vi "Set Bucket Notification.vi"(8 "error in (no error)":errorcluster, 10 "Notification Configuration":T1, 11 "Bucket in":refnum<class "Bucket.lvclass">) -> (0 "error out":errorcluster, 2 "Test Message ID":string, 3 "Bucket out":refnum<class "Bucket.lvclass">)   [LabVIEW 2015, in "NI_AWS_S3.lvlib" / "Bucket.lvclass"]
uses:
  Bucket.lvclass
  Notification Configuration.ctl
  Topic Configuration.ctl
  Event.ctl
  Core/HTTP Request/Name Value Pair.ctl
  Cloud Function Configuration.ctl
  Queue Configuration.ctl
  Core/HTTP Request/Region handling.ctl
  Core/HTTP Request/Request Options.ctl
  Core/HTTP Request/URL formatting.ctl
  Bucket.lvclass/Bucket.ctl
  Read Name.vi
  <vilib>/regexp/Match Regular Expression.xnode
  Core/HTTP Request/HTTP Request.lvclass
  NI_AWS_S3.lvlib
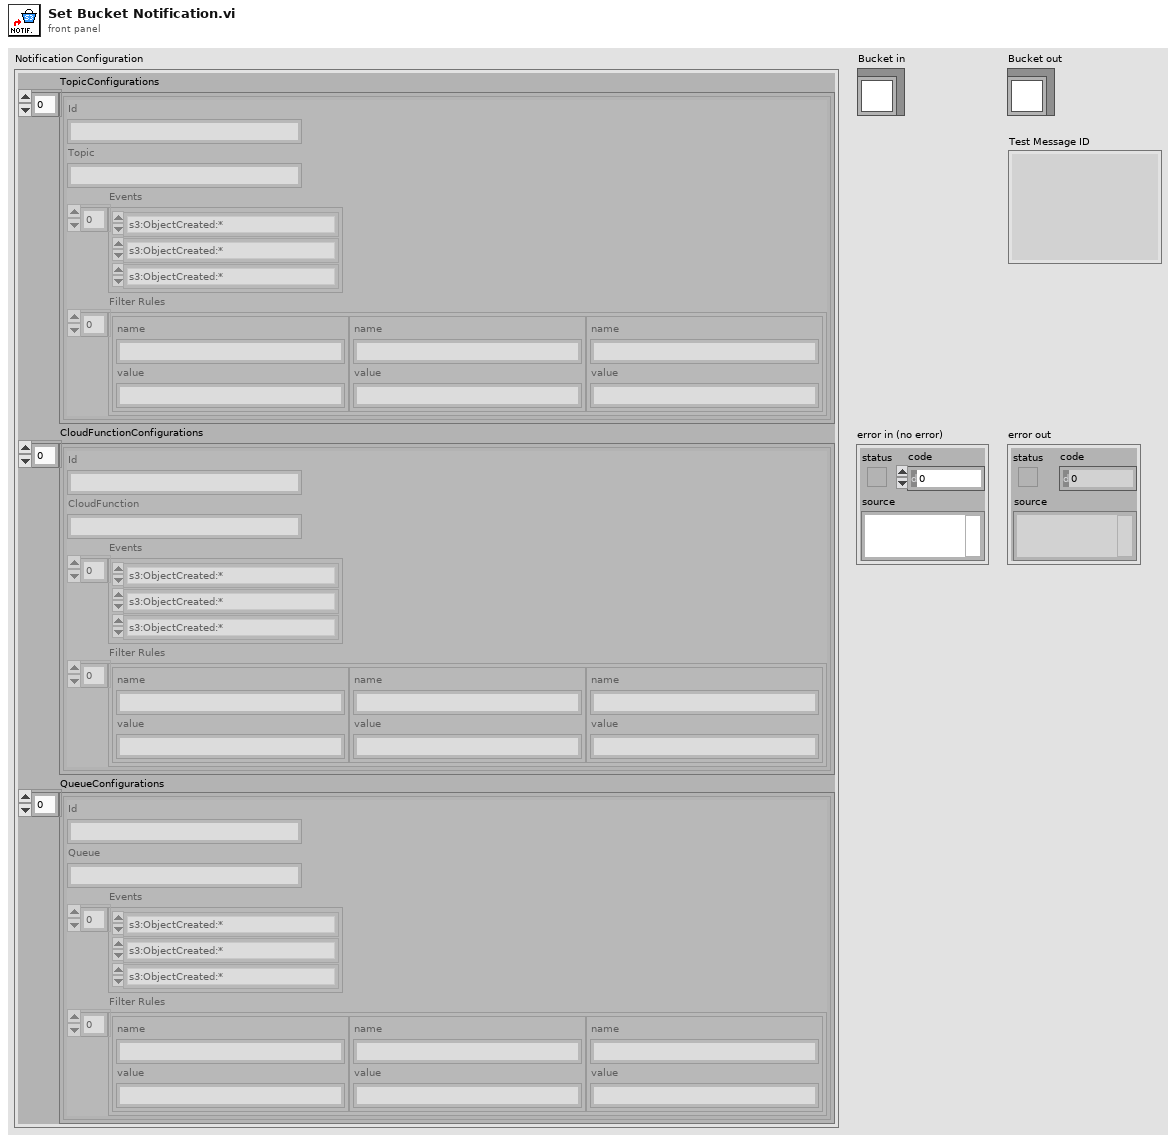
[diagram p1: front panel]
types:
  T1 = typedef "NI_AWS_S3.lvlib/Notification Configuration.ctl" = cluster{"TopicConfigurations":T2[], "CloudFunctionConfigurations":T5[], "QueueConfigurations":T6[]}
  T2 = typedef "NI_AWS_S3.lvlib/Topic Configuration.ctl" = cluster{"Id":string, "Topic":string, "Events":T3[], "Filter Rules":T4[]}
  T3 = typedef "NI_AWS_S3.lvlib/Event.ctl" = enum16{"s3:ObjectCreated:*", "s3:ObjectCreated:Put", "s3:ObjectCreated:Post", "s3:ObjectCreated:Copy", "s3:ObjectCreated:CompleteMultipartUpload", "s3:ObjectRemoved:*", "s3:ObjectRemoved:Delete", "s3:ObjectRemoved:DeleteMarkerCreated", "s3:ReducedRedundancyLostObject"}
  T4 = typedef "NI_AWS_Core.lvlib/HTTP Request.lvclass/Name Value Pair.ctl" = cluster{"name":string, "value":string}
  T5 = typedef "NI_AWS_S3.lvlib/Cloud Function Configuration.ctl" = cluster{"Id":string, "CloudFunction":string, "Events":T3[], "Filter Rules":T4[]}
  T6 = typedef "NI_AWS_S3.lvlib/Queue Configuration.ctl" = cluster{"Id":string, "Queue":string, "Events":T3[], "Filter Rules":T4[]}
  T7 = typedef "NI_AWS_Core.lvlib/HTTP Request.lvclass/Request Options.ctl" = cluster{"request headers":T4[], "request parameters":T4[], "request body":string, "region handling":T8, "URL formatting":T9}
  T8 = typedef "NI_AWS_Core.lvlib/HTTP Request.lvclass/Region handling.ctl" = enum16{"use region everywhere", "use region (authentication only)", "use region (URL only)", "ignore region everwhere"}
  T9 = typedef "NI_AWS_Core.lvlib/HTTP Request.lvclass/URL formatting.ctl" = enum16{"region-", "region."}
  T10 = typedef "NI_AWS_Core.lvlib/HTTP Request.lvclass/Response.ctl" = cluster{"Headers":string, "Body":string}
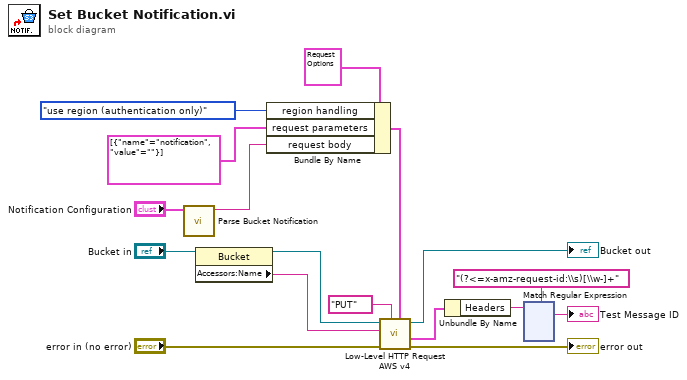
[diagram p0: block diagram]
diagram:
  n1 = call "Parse Bucket Notification.vi"("Notification Parameters"="Notification Configuration") -> ("PUT Data"=w1:string)  [unwired: 10 in]
  n2 = property class="Bucket"(reference="Bucket in") -> (reference out=w9:refnum<class "Bucket.lvclass">, "Accessors:Name"=w17:string)  [unwired: 1 in, 1 out]
  n3 = Bundle By Name(cluster=T7 {"request headers"=[], "request parameters"=[], "request body"="", "region handling"=enum."use region everywhere", "URL formatting"=enum."region."} ("Request Options"), "region handling"=Region_handling."use region (authentication only)", "request parameters"=T4[] [{"name"="notification", "value"=""}], "request body"=w1) -> (w10:T7)
  n4 = call "Low-Level HTTP Request AWS v4.vi"("Request Options"=w10, "HTTP-Verb"="PUT", "error in (no error)"="error in (no error)", "URL Prefix"=w17, "AWS Core in"=w9) -> ("error out"=→"error out":errorcluster, "Response"=w5:T10, "AWS Core out"=→"Bucket out":refnum<class "Bucket.lvclass">)  [unwired: 3 in, 1 out]
  n5 = Unbundle By Name(w5) -> ("Headers"=w4:string)
  n6 = xnode "Match Regular Expression"("input string"=w4, "regular expression"="(?<=x-amz-request-id:\\s)[\\w-]+") -> ("whole match"=→"Test Message ID":string)  [unwired: 4 in, 4 out]
